vi "GreenBoard_ADC_Report_v2.vi"(8 "error in (no error)":errorcluster, 9 "Message IN":string, 10 "Green Board Enum":T1=enum."VLINE_AB", 11 "ControlBoard VISA":refnum<visa-resource-name>="ControlBoard") -> (0 "error out":errorcluster, 1 "Message OUT":string, 2 "Result":dbl, 3 "VISA Refnum out":refnum<visa-resource-name>)   [LabVIEW 2022 SP3]
uses:
  ADCSelector GB.ctl
  SupportVIs/VISA Flush IO Buffer Mask.ctl
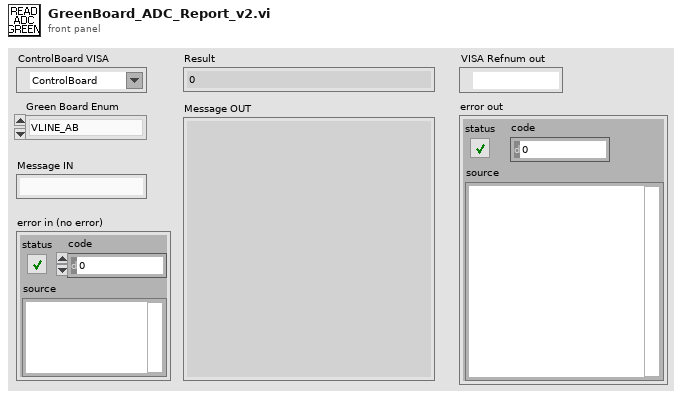
[diagram p1: front panel]
types:
  T1 = typedef "ADCSelector GB.ctl" = enum16{"INVA_ISENSE_U", "INVA_ISENSE_V", "INVA_ISENSE_W", "INVA_UDC", "INVA_TEMP", "HB_ISENSE", "AUX_ISENSE_U", "AUX_ISENSE_V", "AUX_ISENSE_W", "VLINE_AB", "VLINE_BC", "VLINE_CA", "REF_1P5V", "VSENSE_POS_24V", "VSENSE_POS_5V", "VSENSE_NEG_15V", "TEST_POINT", "INVB_ISENSE_U", "INVB_ISENSE_V", "INVB_ISENSE_W", "INVB_UDC", "INVB_TEMP", "HB_TEMP", "AUXA_TEMP", "AUXB_TEMP", "AUXC_TEMP", "VOUT_AB", "VOUT_BC", "VOUT_CA", "REF_2P5V", "VSENSE_POS_15V", "VSENSE_POS_3P3V", "NET_ANALYZER"}
  T2 = typedef "VISA Flush IO Buffer Mask.ctl" = u16
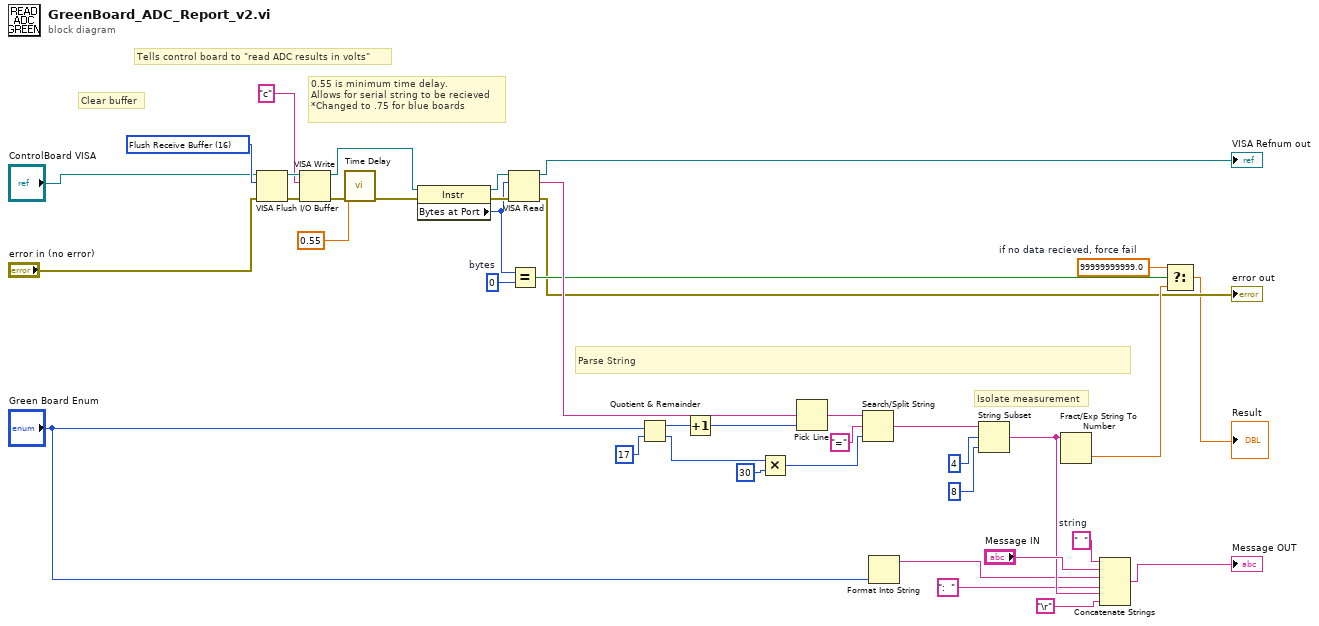
[diagram p0: block diagram]
diagram:
  w10 = "  "  # string
  w16 = 99999999999.0  # if no data recieved, force fail
  w19 = u32 0  # bytes
  w24 = T2 16 items=["Flush Receive Buffer"=16, "Write Transmit Buffer to Device"=32, "Flush Receive Buffer (No I/O)"=64, "Flush Transmit Buffer"=128] ("Mask")
  # "Isolate measurement"
  # "Clear buffer"
  # "Parse String"
  # "0.55 is minimum time delay.\nAllows for serial string to be recieved\n*Changed to .75 for blue boards"
  # "Tells control board to \"read ADC results in volts\""
  n1 = VISA Flush I/O Buffer(VISA resource name="ControlBoard VISA", mask (16)=w24, error in (no error)="error in (no error)") -> (VISA resource name out=w26:refnum<visa-resource-name>, error out=w27:errorcluster)
  n2 = VISA Write(VISA resource name=w26, write buffer="c", error in (no error)=w27) -> (VISA resource name out=w29:refnum<visa-resource-name>, error out=w25:errorcluster)  [unwired: 1 out]
  n3 = call "Time Delay"("error in (no error)"=w25, "Delay Time (s)"=0.55) -> ("error out"=w28:errorcluster)  [unwired: 9 in]
  n4 = property class="Instr"(reference=w29, error in=w28) -> (reference out=w22:refnum<visa-resource-name>, error out=w23:errorcluster, "Bytes at Port"=w20:u32)
  n5 = VISA Read(VISA resource name=w22, byte count=w20, error in (no error)=w23) -> (VISA resource name out=→"VISA Refnum out":refnum<visa-resource-name>, read buffer=w38:string, error out=→"error out":errorcluster)  [unwired: 1 out]
  n6 = Equal?(x=w20, y=w19) -> (x = y?=w17:bool)
  n7 = Quotient & Remainder(x="Green Board Enum", y=17) -> (x-y*floor(x/y)=w33:i32, floor(x/y)=w35:i32)
  n8 = Increment(x=w33) -> (x+1=w34:i32)
  n9 = Multiply(x=w35, y=30) -> (x*y=w37:i32)
  n10 = Pick Line(multi-line string=w38, line index=w34) -> (output string=w39:string)  [unwired: 1 in]
  n11 = Search/Split String(string=w39, search string/char (-)="=" ("regular expression"), offset (0)=w37) -> (match + rest of string=w31:string)  [unwired: 2 out]
  n12 = Format Into String("Green Board Enum") -> (resulting string=w3:string)  [unwired: 3 in, 1 out]
  n13 = String Subset(string=w31, offset (0)=4, length (rest)=8 ("offset (0)")) -> (substring=w12:string)
  n14 = Fract/Exp String To Number(string=w12) -> (number=w18:dbl)  [unwired: 3 in, 1 out]
  n15 = Concatenate Strings(w10, "Message IN", w3, ":  ", w12, "\r") -> (→"Message OUT":string)
  n16 = Select(t=w16, s=w17, f=w18) -> (s? t:f=→"Result":dbl)
